vi "U3 DAC_Kevin_MFC_PID_flow.vi"() -> ()   [LabVIEW 2016]
uses:
  OdorSensorArray/labview 2016 code/osa_global_save2.vi
  <vilib>/Utility/file.llb/Read From Spreadsheet File (DBL).vi
  <vilib>/measure/NI_MABase.lvlib
panel:
  in  "Stair interval (s)":u32=20
  out "Error U3-2 A0":string
  out "PID / flow":cluster{"Value Read":dbl, "Value Read":dbl}(graph)
  in  "Dilusion_DACB":dbl step=0.1 format="%.4f"
  out "elapsed time":string="00:00:00.000"
  in  "MFC_sequence":path
  out "Array Size":i32
  out "Udate Array from File":sgl[](array[numeric])
  out "Error  PID_Save":string
  out "error write":errorcluster
  in  "Save file":bool
  in  "save data folder":path
  out "appended path":path
  out "AIN0":dbl format="%.6f"
  out "MFC I/O":cluster{"Value Read":dbl, "Value Read":dbl}(graph)
  out "AIN2":dbl format="%.6f"
  out "AIN1":dbl format="%.6f"
  in  "DAC0_type":enum16{"functional", "fixed", "read"}(ring)
  out "Waveform Chart":dbl(graph)
  in  "DAC0_fixed":dbl step=0.1 format="%.4f"
  out "Error DAC1,B":string
  out "error read":errorcluster
  in  "Background_DAC1":dbl step=0.1 format="%.4f"
  in  "Update Interval (ms)":u32=20
  out "Error_DAC0":string
  in  "Function":u16(ring) items=["Sine Wave", "Triangle Wave", "Square Wave", "Sawtooth Wave"]
  in  "Min Voltage":dbl=0.5 min=0.0 max=5.0 step=0.1 format="%.2f"
  in  "Max Voltage":dbl=4.5 min=0.0 max=5.0 step=0.1 format="%.2f"
  in  "Frequency (Hz)":dbl=1.0 step=0.1 format="%.3f"
  in  "Stop":bool
  # "Updates DAC0 at the specified update interval in order to build time series waveforms.  The\nupdate interval is set to 20 ms by default, but can be set lower based on the execution times\ndiscussed in Section 3.1 of the U3 User's Guide.  Uses the first found U3.\n\nWith a software timed application such as this, you might be able to reduce timing jitter (caused\nby the operating system) by increasing the priority of this process (labview.exe) in Windows\nTask Manager."
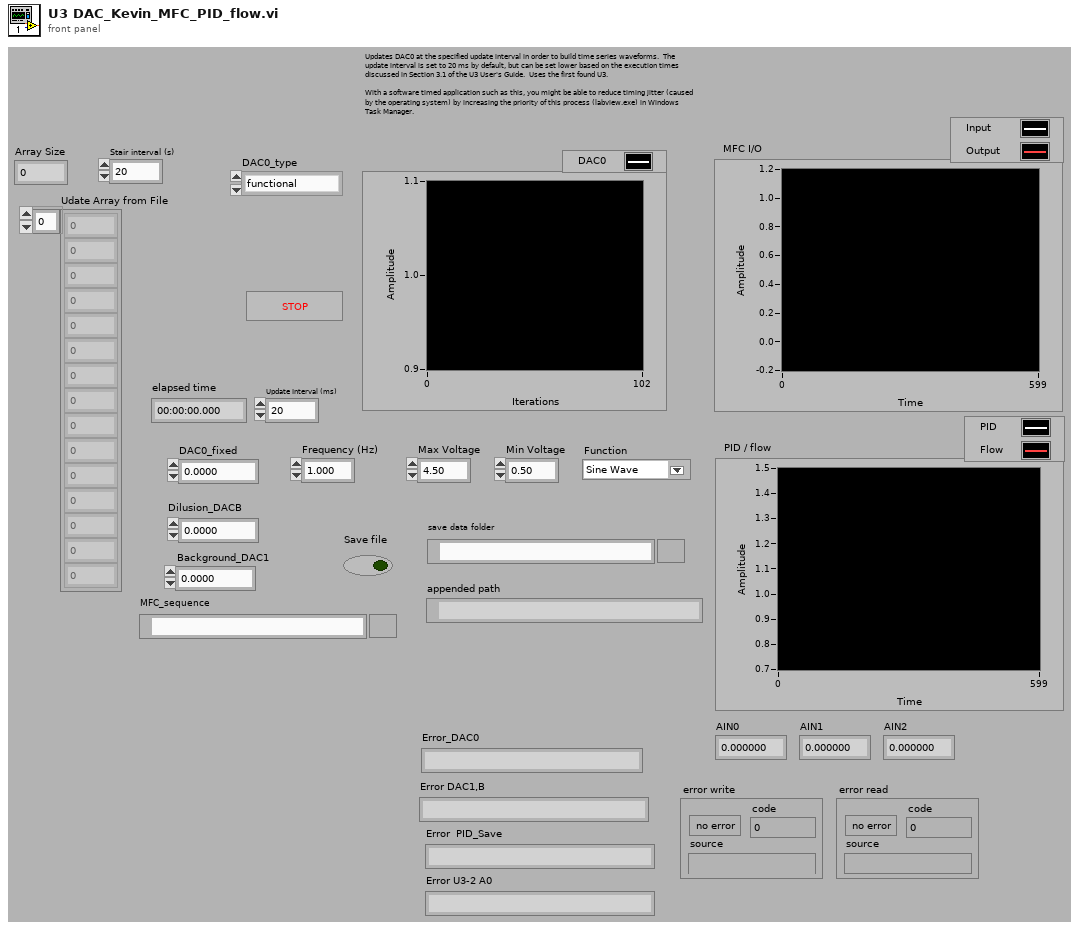
[diagram p1: front panel]
types:
  T1 = enum16{"open", "replace", "create", "open or create", "replace or create", "replace or create with confirmation"}
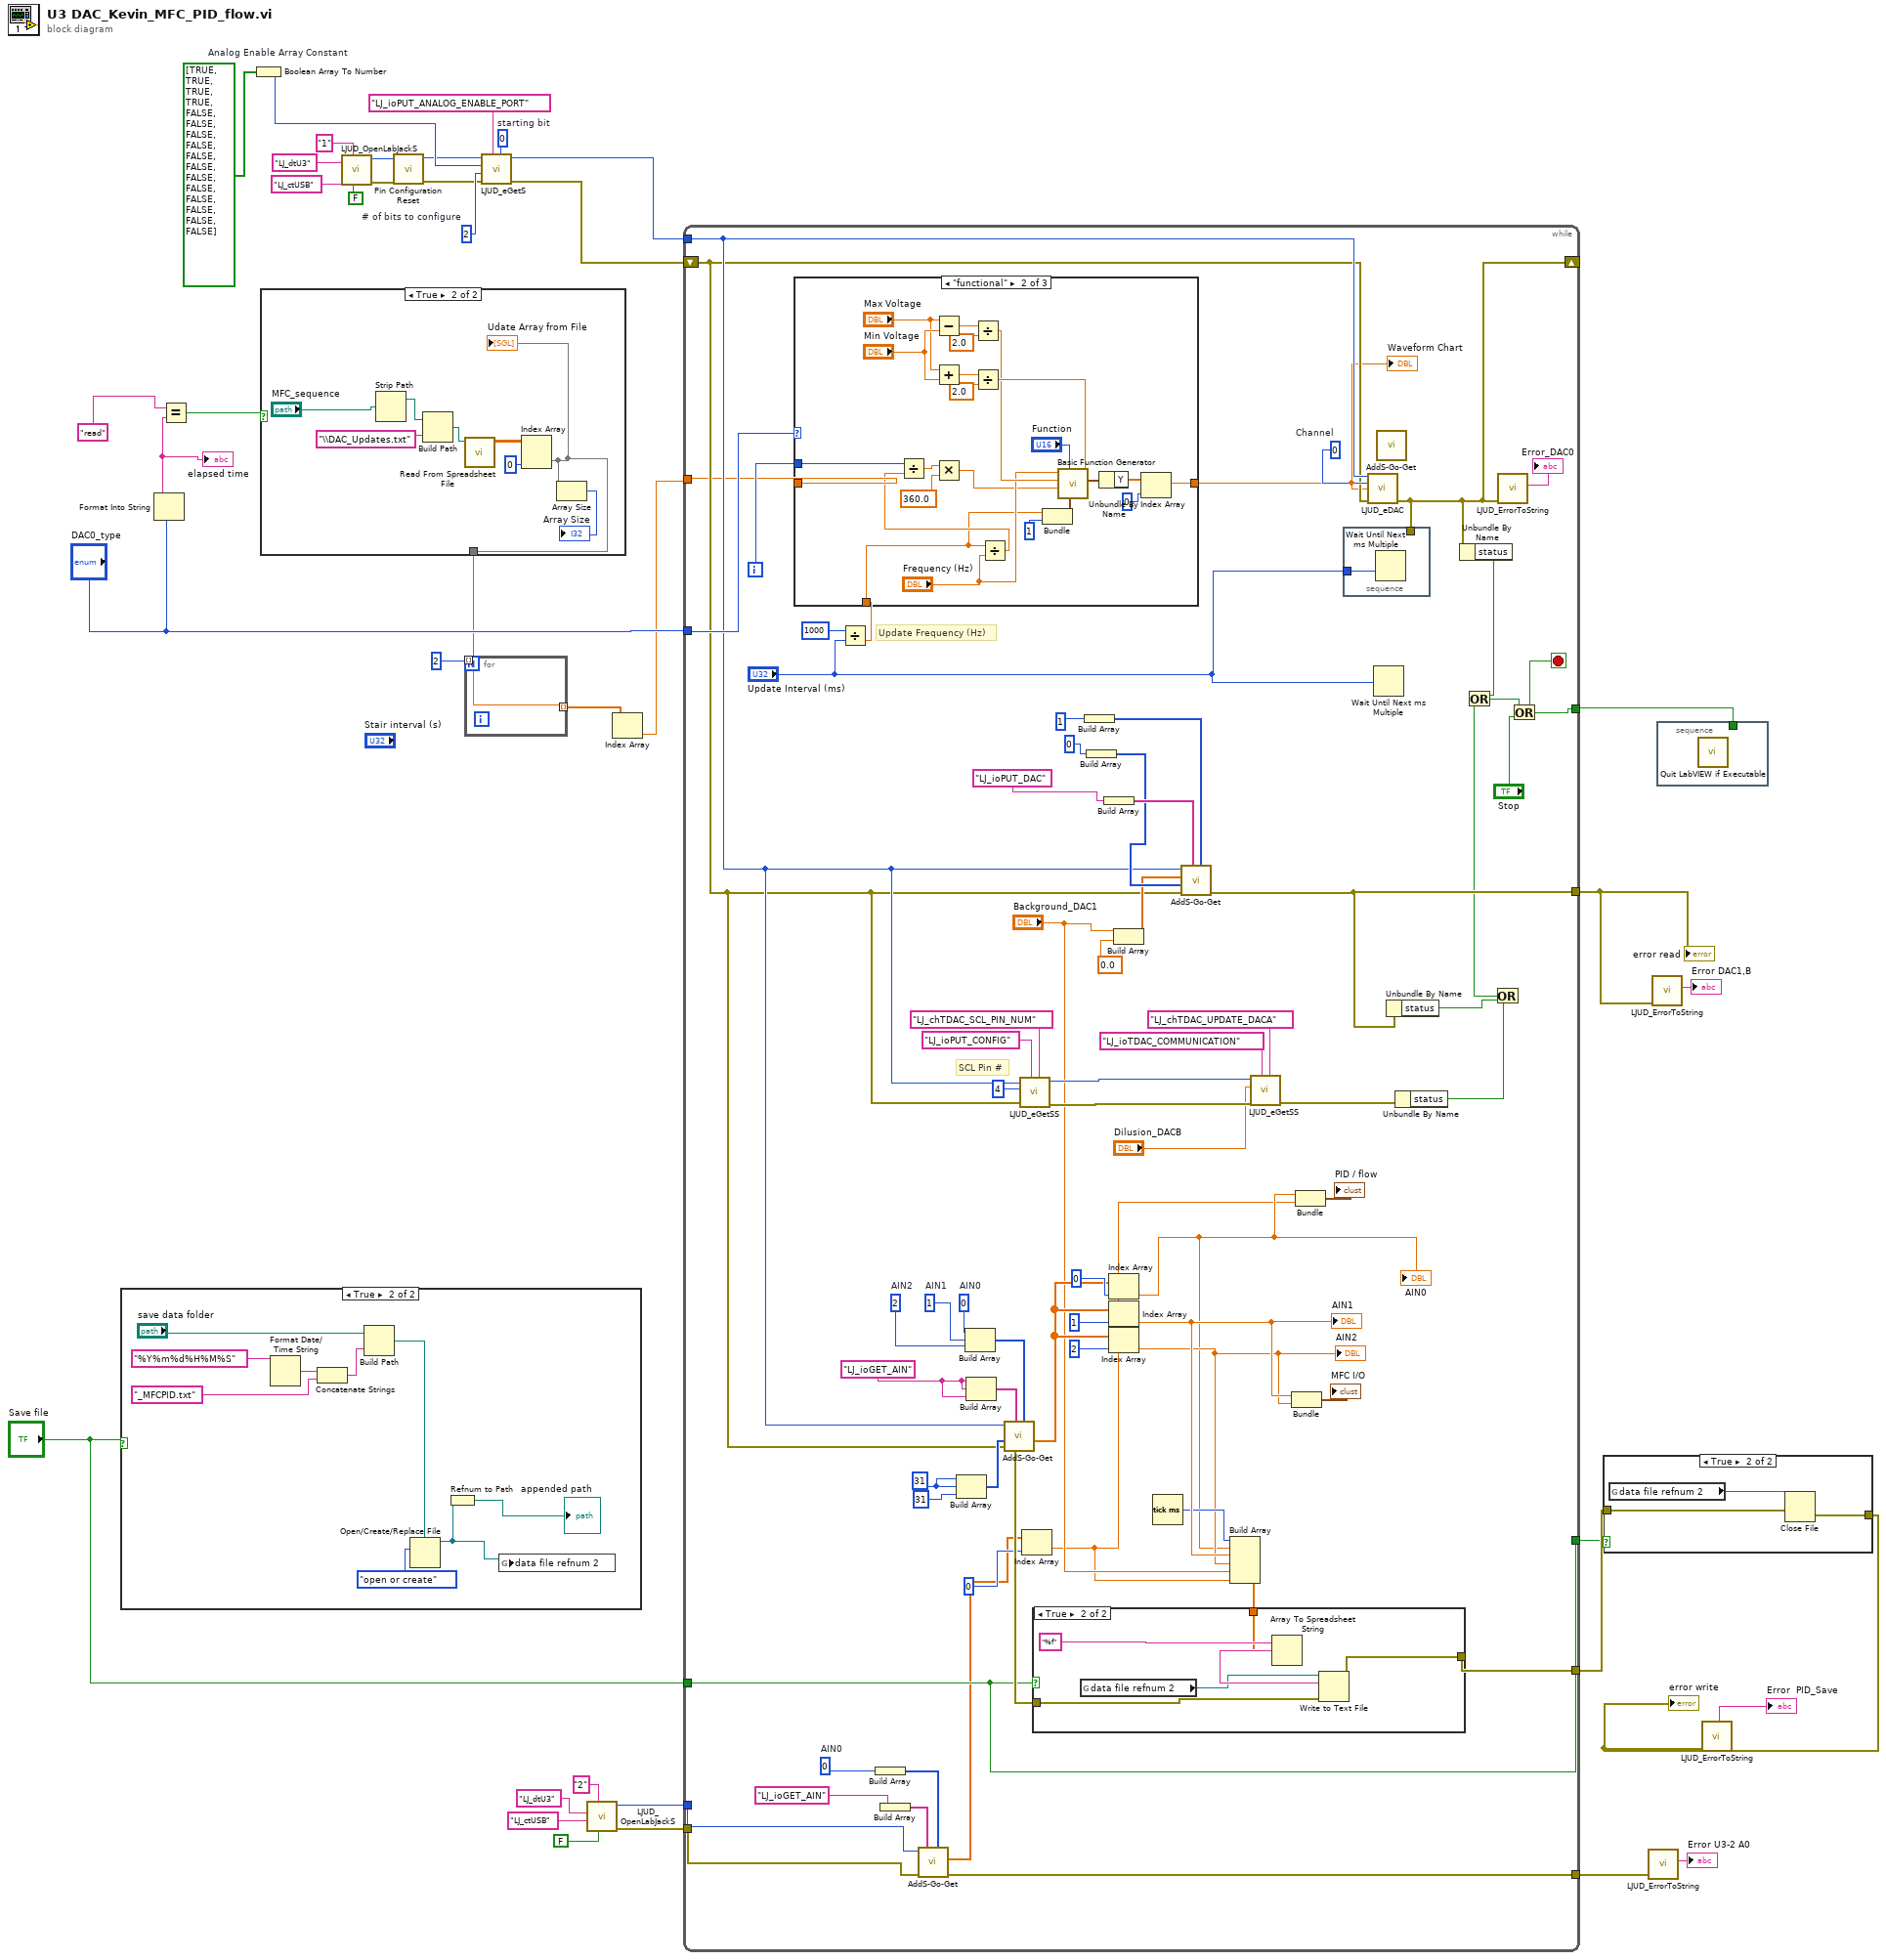
[diagram p0: block diagram]
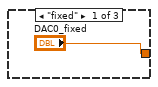
[diagram p6: hidden frame]
diagram:
  w27 = 2  # # of bits to configure
  w29 = 0  # starting bit
  w30 = bool[] [TRUE, TRUE, TRUE, TRUE, FALSE, FALSE, FALSE, FALSE, FALSE, FALSE, FALSE, FALSE, FALSE, FALSE, FALSE, FALSE]  # Analog Enable Array Constant
  n1 = case shown="True" "Save file" {
    frame False {
    }
    frame True {
      n2 = Format Date/Time String(time format string (%c)="%Y%m%d%H%M%S") -> (date/time string=w45:string)  [unwired: 2 in]
      n3 = Concatenate Strings(w45, "_MFCPID.txt") -> (w47:string)
      n4 = Build Path(base path="save data folder", name or relative path=w47) -> (appended path=w41:path)
      n5 = Open/Create/Replace File(file path (use dialog)=w41, operation (0:open)=T1."open or create") -> (refnum out=w40:refnum<file>)  [unwired: 4 in, 2 out]
      n6 = Refnum to Path(1:w40) -> (0:→"appended path":path)
      n7 = global write "osa_global_save2.vi" "data file refnum 2"(w40) -> ()
    }
  }
  n8 = Format Into String("DAC0_type") -> (resulting string=w13:string)  [unwired: 3 in, 1 out]
  "elapsed time" <- w13
  n9 = Equal?(x="read", y=w13) -> (x = y?=w16:bool)
  n10 = Boolean Array To Number(Boolean array=w30) -> (number=w26:u32)
  n11 = case shown="True" w16 {
    tunnel: [_ w49] -> w2
    frame False {
    }
    frame True {
      n12 = Strip Path(path="MFC_sequence") -> (stripped path=w51:path)  [unwired: 1 out]
      n13 = Build Path(base path=w51, name or relative path="\\DAC_Updates.txt" ("file path (dialog if empty)")) -> (appended path=w52:path)
      n14 = call-poly <vilib>:"Read From Spreadsheet File.vi"("file path (dialog if empty)"=w52) -> ("all rows"=w56:dbl[][])  [unwired: 6 in, 4 out]
      n15 = Index Array(array=w56, index (col)=0 ("disabled index (col)")) -> (element=w49:dbl[])  [unwired: 1 in]
      "Udate Array from File" <- w49
      n16 = Array Size(array=w49) -> (size(s)=→"Array Size":i32)
    }
  }
  n17 = call "LJUD_OpenLabJackS.vi"("FirstFound"=FALSE, "Address"="1" ("DeviceType"), "ConnectionType"="LJ_ctUSB", "DeviceType"="LJ_dtU3") -> ("error out"=w31:errorcluster, "Handle"=w32:i32)  [unwired: 5 in, 1 out]
  n18 = call "Pin Configuration Reset.vi"("error in"=w31, "Handle In"=w32) -> ("error out"=w24:errorcluster, "Handle Out"=w25:i32)  [unwired: 8 in]
  n19 = for {
    N: u32 2 ("x") -> [_]
    tunnel: [w57] -> w3 mode=indexing
    tunnel: w2 -> [w57] mode=indexing
  }
  n20 = call "LJUD_eGetS.vi"("Channel"=w29, "IOType"="LJ_ioPUT_ANALOG_ENABLE_PORT", "error in"=w24, "x1"=w27, "Value Write"=w26, "Handle In"=w25) -> ("error out"=w22:errorcluster, "Handle Out"=w23:i32)  [unwired: 3 in, 1 out]
  n21 = call "LJUD_OpenLabJackS.vi"("FirstFound"=FALSE, "Address"="2", "ConnectionType"="LJ_ctUSB", "DeviceType"="LJ_dtU3") -> ("error out"=w7:errorcluster, "Handle"=w8:i32)  [unwired: 5 in, 1 out]
  n22 = Index Array(array=w3) -> (element=w1:dbl)  [unwired: 1 in]
  n23 = while {
    tunnel: w23 -> [w81]
    shift-left: w22 -> [w80]
    shift-right: [w124] -> _
    tunnel: [w110] -> w39
    tunnel: [w113] -> w37
    tunnel: "DAC0_type" -> [w109]
    tunnel: w1 -> [w58]
    tunnel: [w77] -> w21
    tunnel: "Save file" -> [w75]
    tunnel: [w75] -> w19
    tunnel: w8 -> [w67]
    tunnel: w7 -> [w66]
    tunnel: [w61] -> w5
    i -> [w128]
    stop <- w110 stop-if-true
    w70 = 0  # AIN0
    w87 = 2  # AIN2
    w83 = 31 ("AIN0")
    w92 = 1  # AIN1
    w91 = 0  # AIN0
    w84 = "LJ_ioGET_AIN" ("IOType")
    w125 = 0  # Channel
    # "SCL Pin #"
    # "Update Frequency (Hz)"
    n24 = Divide(x=u32 1000, y="Update Interval (ms)") -> (x/y=w122:dbl)
    n25 = case shown="\"functional\"" w109 {
      tunnel: w128 -> [_ w158 _]
      tunnel: ["DAC0_fixed" w138 w159] -> w59
      tunnel: w122 -> [_ w137 _]
      tunnel: w58 -> [_ _ w159]
      frame "fixed" {
      }
      frame "functional" {
        n26 = Subtract(x="Max Voltage", y="Min Voltage") -> (x-y=w155:dbl)
        n27 = Add(x="Max Voltage", y="Min Voltage") -> (x+y=w152:dbl)
        n28 = Divide(x=w155, y=2.0) -> (x/y=w147:dbl)
        n29 = Divide(x=w152, y=2.0) -> (x/y=w148:dbl)
        n30 = Divide(x=w137, y="Frequency (Hz)") -> (x/y=w157:dbl)
        n31 = Divide(x=w158, y=w157) -> (x/y=w156:dbl)
        n32 = Multiply(x=w156, y=360.0) -> (x*y=w144:dbl)
        n33 = Bundle(w137, 1) -> (w142:cluster{dbl, i32})  [unwired: 1 in]
        n34 = call <vilib>:"Basic Function Generator.vi"("offset"=w148, "sampling info"=w142, "signal type"="Function", "phase"=w144, "amplitude"=w147, "frequency"="Frequency (Hz)") -> ("signal out"=w141:waveform(dbl))  [unwired: 3 in, 2 out]
        n35 = Unbundle By Name(w141) -> ("Y"=w140:dbl[])
        n36 = Index Array(array=w140, index=0 ("Index")) -> (element=w138:dbl)
      }
      frame "read" {
      }
    }
    "Waveform Chart" <- w59
    n37 = Build Array(w70) -> (w71:i32[])
    n38 = Build Array("LJ_ioGET_AIN" ("IOType")) -> (w69:string[])
    n39 = call "AddS-Go-Get.vi"("Channels"=w71, "IOTypes"=w69, "error in"=w66, "Handle In"=w67) -> ("error out"=w61:errorcluster, "Values Read"=w62:dbl[])  [unwired: 5 in, 1 out]
    n40 = Build Array(w83, w83, 31 ("AIN1")) -> (w88:i32[])
    n41 = Build Array(w91, w92, w87) -> (w95:i32[])
    n42 = Build Array(w84, w84, w84) -> (w96:string[])
    n43 = call "AddS-Go-Get.vi"("Channels"=w95, "IOTypes"=w96, "error in"=w80, "x1"=w88, "Handle In"=w81) -> ("error out"=w78:errorcluster, "Values Read"=w76:dbl[])  [unwired: 4 in, 1 out]
    n44 = call "LJUD_eGetSS.vi"("Channel"="LJ_chTDAC_SCL_PIN_NUM", "IOType"="LJ_ioPUT_CONFIG", "error in"=w80, "Value Write"=4, "Handle In"=w81) -> ("error out"=w97:errorcluster, "Handle Out"=w98:i32)  [unwired: 4 in, 1 out]
    n45 = Index Array(array=w62, index=0 ("Index")) -> (element=w60:dbl)
    n46 = Build Array(1) -> (w120:i32[])
    n47 = Build Array(0) -> (w115:i32[])
    n48 = Build Array("LJ_ioPUT_DAC" ("IOType")) -> (w121:string[])
    n49 = Index Array(array=w76, index=0 ("Index")) -> (element=w64:dbl)
    "AIN0" <- w64
    n50 = Index Array(array=w76, index=1 ("Index")) -> (element=w85:dbl)
    "AIN1" <- w85
    n51 = Index Array(array=w76, index=2 ("Index")) -> (element=w79:dbl)
    "AIN2" <- w79
    n52 = Build Array("Background_DAC1", 0.0 ("Input Element")) -> (w105:dbl[])
    n53 = Tick Count (ms)() -> (millisecond timer value=w82:u32)
    n54 = call "AddS-Go-Get.vi"("Channels"=w120, "IOTypes"=w121, "error in"=w80, "x1"=w115, "Values Write"=w105, "Handle In"=w81) -> ("error out"=w113:errorcluster)  [unwired: 3 in, 2 out]
    n55 = Build Array(w82, w64, w85, w79, "Background_DAC1", w60) -> (w74:dbl[])
    n56 = case shown="True" w75 {
      tunnel: w78 -> [w129 w134]
      tunnel: [w129 w133] -> w77
      tunnel: w74 -> [_ w130]
      frame False {
      }
      frame True {
        n57 = global read "osa_global_save2.vi" "data file refnum 2"() -> (w131:refnum<file>)
        n58 = Array To Spreadsheet String(array=w130, 3:"%f") -> (spreadsheet string=w132:string)  [unwired: 1 in]
        n59 = Write to Text File(file (use dialog)=w131, text=w132, error in=w134) -> (error out=w133:errorcluster)  [unwired: 1 in, 2 out]
      }
    }
    n60 = call "LJUD_eGetSS.vi"("Channel"="LJ_chTDAC_UPDATE_DACA", "IOType"="LJ_ioTDAC_COMMUNICATION", "error in"=w97, "Value Write"="Dilusion_DACB", "Handle In"=w98) -> ("error out"=w99:errorcluster)  [unwired: 4 in, 2 out]
    n61 = Bundle("Value Read"=w85, "Value Read"=w79) -> (→"MFC I/O":cluster{"Value Read":dbl, "Value Read":dbl})  [unwired: 1 in]
    n62 = Bundle("Value Read"=w64, "Value Read"=w60) -> (→"PID / flow":cluster{"Value Read":dbl, "Value Read":dbl})  [unwired: 1 in]
    n63 = call "LJUD_eDAC.vi"("Handle In"=w81, "Channel"=w125, "Voltage"=w59, "error in"=w80) -> ("error out"=w124:errorcluster)  [unwired: 10 in, 1 out]
    n64 = stacked-sequence {
      tunnel: "Update Interval (ms)" -> [w160]
      tunnel: w124 -> [_]
      frame #0 {
        n65 = Wait Until Next ms Multiple(millisecond multiple=w160) -> ()  [unwired: 1 out]
      }
    }
    n66 = Wait Until Next ms Multiple(millisecond multiple="Update Interval (ms)") -> ()  [unwired: 1 out]
    n67 = call "AddS-Go-Get.vi"() -> ()  [unwired: 9 in, 3 out]
    n68 = Unbundle By Name(w113) -> ("status"=w102:bool)
    n69 = Unbundle By Name(w99) -> ("status"=w103:bool)
    n70 = Unbundle By Name(w124) -> ("status"=w112:bool)
    n71 = Or(x=w103, y=w102) -> (x .or. y?=w104:bool)
    n72 = Or(x=w112, y=w104) -> (x .or. y?=w111:bool)
    n73 = call "LJUD_ErrorToString.vi"("error in"=w124) -> ("String"=→"Error_DAC0":string)  [unwired: 10 in]
    n74 = Or(x=w111, y="Stop") -> (x .or. y?=w110:bool)
  }
  "error read" <- w37
  n75 = case shown="True" w19 {
    tunnel: w21 -> [w161 w164]
    tunnel: [w161 w163] -> w17
    frame False {
    }
    frame True {
      n76 = global read "osa_global_save2.vi" "data file refnum 2"() -> (w162:refnum<file>)
      n77 = Close File(refnum=w162, error in=w164) -> (error out=w163:errorcluster)  [unwired: 1 out]
    }
  }
  "error write" <- w17
  n78 = call "LJUD_ErrorToString.vi"("error in"=w5) -> ("String"=→"Error U3-2 A0":string)  [unwired: 10 in]
  n79 = call "LJUD_ErrorToString.vi"("error in"=w37) -> ("String"=→"Error DAC1,B":string)  [unwired: 10 in]
  n80 = stacked-sequence {
    tunnel: w39 -> [_]
    frame #0 {
      n81 = call "Quit LabVIEW if Executable.vi"() -> ()  [unwired: 1 in]
    }
  }
  n82 = call "LJUD_ErrorToString.vi"("error in"=w17) -> ("String"=→"Error  PID_Save":string)  [unwired: 10 in]
